vi "Read Save Timestamp.vi"(8 "error in (no error)":errorcluster, 11 "File in":refnum<class "File.lvclass">) -> (0 "error out":errorcluster, 2 "Save Timestamp":bool, 3 "File out":refnum<class "File.lvclass">)   [LabVIEW 2020, in "Manejador archivo.lvlib" / "File.lvclass"]
uses:
  File.lvclass
  File.lvclass/File.ctl
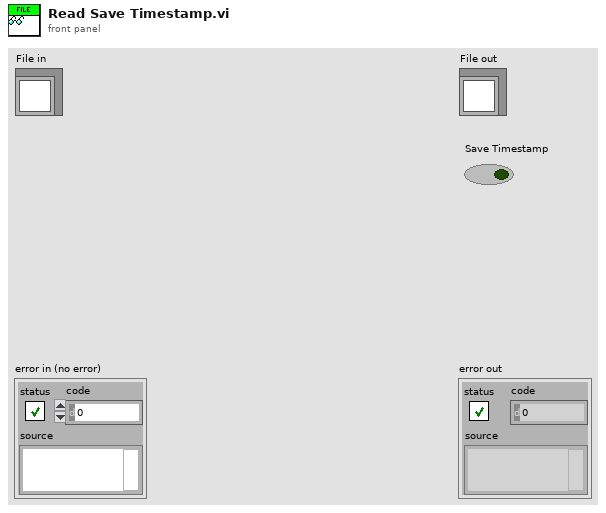
[diagram p1: front panel]
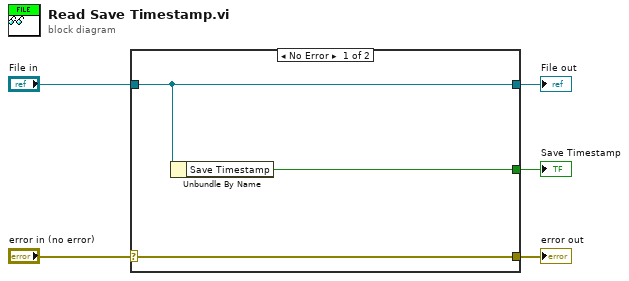
[diagram p0: block diagram]
diagram:
  n1 = case shown="No Error" "error in (no error)" {
    selector: "error in (no error)" -> [w8 w9]
    tunnel: [w8 w9] -> w4
    tunnel: [w7 w10] -> w2
    tunnel: "File in" -> [w7 w10]
    tunnel: [w6 _] -> w1
    frame No Error {
      n2 = Unbundle By Name(w7) -> ("Save Timestamp"=w6:bool)
    }
    frame Error {
    }
  }
  "error out" <- w4
  "File out" <- w2
  "Save Timestamp" <- w1
